vi "Windows run ipconfig.vi"(8 "error in (no error)":errorcluster) -> (0 "error out":errorcluster, 3 "standard output":string)   [LabVIEW 2020, in "NI_WFCN.lvlib" / "Hostname Network Address.lvclass"]
doc: "Windows: Run `ipconfig` to identify configured DNS servers."
uses:
  <vilib>/net/WFCN/Addressing/Hostname Network Address/Hostname Network Address.lvclass
  <vilib>/net/WFCN/NI_WFCN.lvlib
panel:
  out "standard error":string
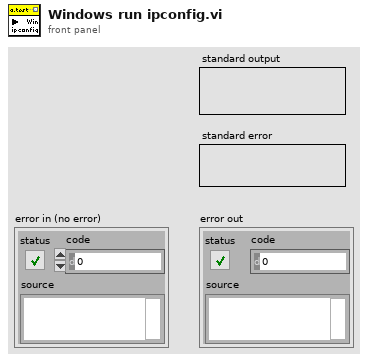
[diagram p1: front panel]
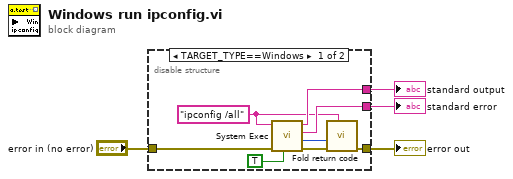
[diagram p0: block diagram]
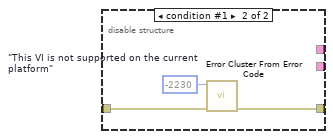
[diagram p2: hidden frame]
diagram:
  n1 = disable-structure shown="TARGET_TYPE==Windows" {
    disable-tunnel: [w7 w13] -> w4
    disable-tunnel: "error in (no error)" -> [w12 w14]
    disable-tunnel: [w11 _] -> w2
    disable-tunnel: [w9 _] -> w1
    frame condition #0 (active) {
      w6 = "ipconfig /all" ("command line")
      n2 = call <vilib>:"System Exec.vi"("run minimized? (F)"=TRUE, "error in (no error)"=w12, "command line"=w6) -> ("error out"=w8:errorcluster, "return code"=w5:i32, "standard error"=w9:string, "standard output"=w11:string)  [unwired: 5 in]
      n3 = call <vilib>:"Fold return code.vi"("command"=w6, "error in (no error)"=w8, "return code"=w5) -> ("error out"=w7:errorcluster)  [unwired: 8 in]
    }
    frame condition #1 {
      w15 = -2230  # "This VI is not supported on the current platform"
      n4 = call <vilib>:"Error Cluster From Error Code.vi"("error in (no error)"=w14, "error code (0)"=w15) -> ("error out"=w13:errorcluster)  [unwired: 7 in]
    }
  }
  "error out" <- w4
  "standard output" <- w2
  "standard error" <- w1
